vi "CreateLogFolder.vi"(11 "Base Folder":path=path "E:/maggot images/Jacob") -> (0 "error out":errorcluster, 3 "Path Out":path)   [LabVIEW 2016]
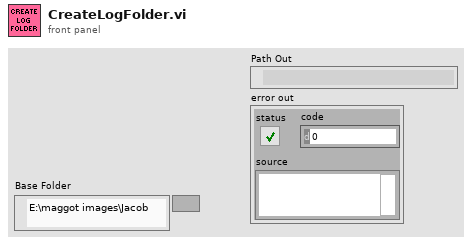
[diagram p1: front panel]
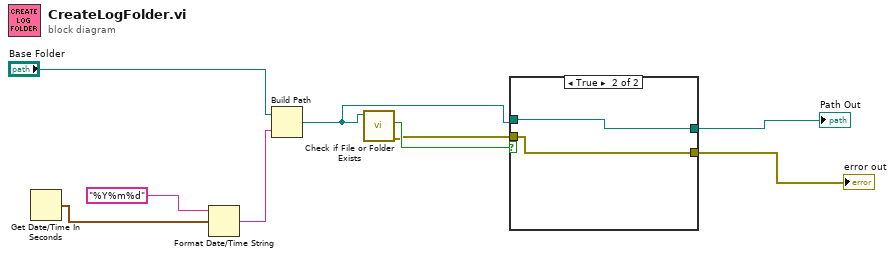
[diagram p0: block diagram]
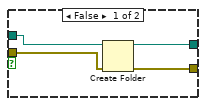
[diagram p2: hidden frame]
diagram:
  n1 = Get Date/Time In Seconds() -> (seconds since 1Jan1904=w9:timestamp)
  n2 = Format Date/Time String(time format string (%c)="%Y%m%d", seconds (now)=w9) -> (date/time string=w7:string)  [unwired: 1 in]
  n3 = Build Path(base path="Base Folder", name or relative path=w7) -> (appended path=w1:path)
  n4 = call <vilib>:"Check if File or Folder Exists.vi"("path"=w1) -> ("error out"=w4:errorcluster, "file or folder exists?"=w5:bool)  [unwired: 8 in, 1 out]
  n5 = case shown="True" w5 {
    tunnel: w4 -> [w13 w14]
    tunnel: [w12 w14] -> w2
    tunnel: [w11 w15] -> w3
    tunnel: w1 -> [w10 w15]
    frame False {
      n6 = Create Folder(path (use dialog)=w10, error in=w13) -> (created path=w11:path, error out=w12:errorcluster)  [unwired: 1 in, 1 out]
    }
    frame True {
    }
  }
  "Path Out" <- w3
  "error out" <- w2
